vi "Test_InsertAndRemoveViewModel_NoError.vi"(8 "error in (no error)":errorcluster, 11 "TestCase in":refnum<class "TestIViewModel.lvclass">) -> (0 "error out":errorcluster, 3 "TestCase out":refnum<class "TestIViewModel.lvclass">)   [LabVIEW 2017, in "TestIViewModel.lvclass"]
uses:
  TestIViewModel.lvclass
  Framework/IViewModel/IViewModel/IViewModel.lvclass
  C:/Git/mva-framework/Framework/IViewManager/IViewManager/IViewManager.lvclass
  C:/Program Files (x86)/National Instruments/LabVIEW 2017/vi.lib/ActorFramework/Actor/Actor.lvclass
  Doubles/ViewableDoubles/ViewableOne/ViewableOne.lvclass
  C:/Git/mva-framework/Framework/IViewable/IViewable/IViewable.lvclass
  Framework/IModel/IModel/IModel.lvclass
  Framework/Mediator/Mediator/Mediator.lvclass
  C:/Git/mva-framework/Framework/IMediator/IMediator/IMediator.lvclass
  Framework/IViewModel/IViewModel/IViewModel.lvclass/IViewModel.ctl
  Framework/IViewManager/IViewManager Messages/Launch Nested Views Msg/Launch Nested Views Msg.lvclass/Launch Nested Views Msg.ctl
  Framework/IViewManager/IViewManager/IViewManager.lvclass/IViewManager.ctl
  Framework/IViewable/IViewable Messages/Insert Front Panel Msg/Insert Front Panel Msg.lvclass/Insert Front Panel Msg.ctl
  <vilib>/ActorFramework/Message Enqueuer/Message Enqueuer.lvclass/Message Enqueuer.ctl
  Framework/IViewable/IViewable Messages/Close Front Panel Msg/Close Front Panel Msg.lvclass/Close Front Panel Msg.ctl
  Framework/IViewManager/IViewManager Messages/Launch Nested Views Msg/Pack Launch Nested Views Msg.vi
  Framework/IViewManager/IViewManager/Write Startup Launch Nested Views Msg.vi
  <vilib>/ActorFramework/Message Enqueuer/Enqueue.vi
  Framework/IViewable/IViewable Messages/Insert Front Panel Msg/Insert Front Panel Msg.lvclass
  C:/Program Files (x86)/National Instruments/LabVIEW 2017/vi.lib/ActorFramework/Message/Message.lvclass
  Framework/IViewable/IViewable Messages/Close Front Panel Msg/Close Front Panel Msg.lvclass
  <vilib>/ActorFramework/Stop Msg/Stop Msg.lvclass
  <vilib>/ActorFramework/Message Priority Queue/Priority Enqueue.vi
  Framework/IViewable/IApplicationStyle/IApplicationStyle.lvclass
  Framework/IViewManager/IViewManager Messages/Launch Nested Views Msg/Launch Nested Views Msg.lvclass
  <vilib>/ActorFramework/Actor/Actor.lvclass
  Framework/IViewable/ProtectedSubpanel/ProtectedSubpanel.lvclass
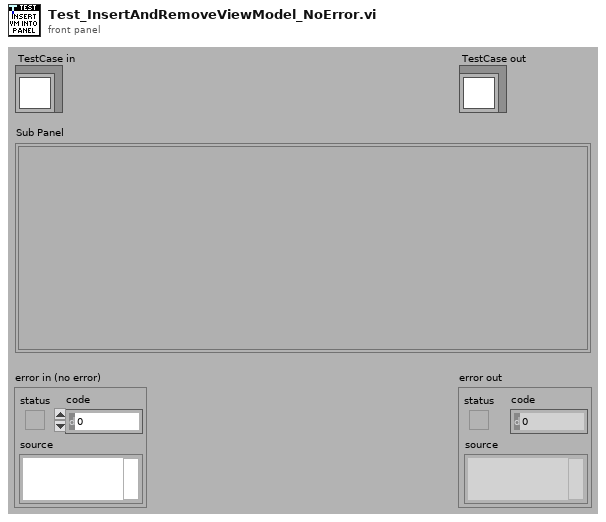
[diagram p1: front panel]
types:
  T1 = typedef "IViewable.lvlib/ProtectedSubpanel.lvclass/Protected Subpanel Reference.ctl" = refnum<data-value>
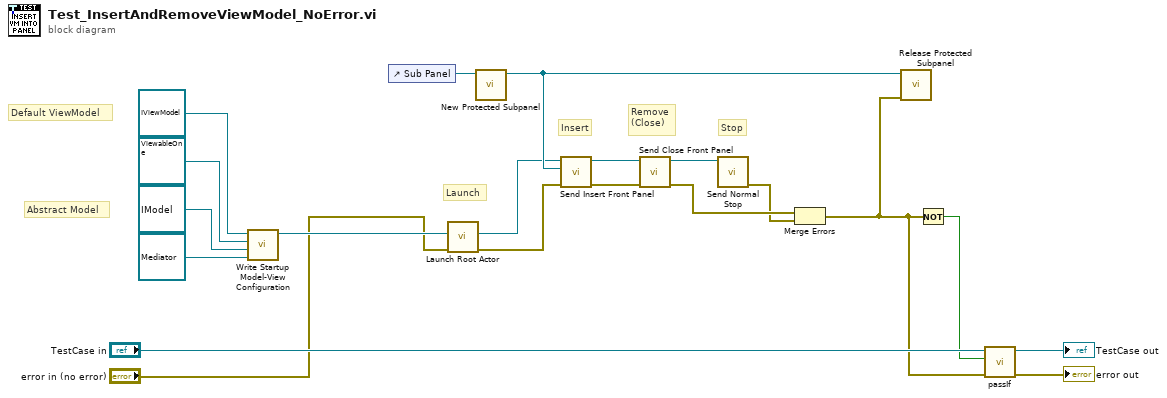
[diagram p0: block diagram]
diagram:
  # "Remove\n(Close)"
  # "Insert"
  # "Stop"
  # "Launch"
  # "Abstract Model"
  # "Default ViewModel"
  n1 = call "Write Startup Model-View Configuration.vi"("Mediator Type"=refnum<class "Mediator.lvclass"> refnum ("Mediator"), "Model Type"=refnum<class "IModel.lvclass"> refnum ("Model"), "Startup View Configuration"=refnum<class "ViewableOne.lvclass"> refnum, "IViewModel In"=refnum<class "IViewModel.lvclass"> refnum) -> ("IViewModel Out"=w12:refnum<class "IViewModel.lvclass">)  [unwired: 7 in]
  n2 = control-ref of="Sub Panel"() -> (w10:refnum<vi>)
  n3 = call <vilib>:"Launch Root Actor.vi"("error in (no error)"="error in (no error)", "Actor"=w12) -> ("error out"=w6:errorcluster, "Actor's Enqueuer"=w7:refnum<class "Message Enqueuer.lvclass">)  [unwired: 8 in]
  n4 = call "New Protected Subpanel.vi"("SubPnl Refnum"=w10) -> ("Protected Subpanel"=w9:T1)  [unwired: 9 in, 1 out]
  n5 = call "Send Insert Front Panel.vi"("error in (no error)"=w6, "Protected Subpanel"=w9, "Message Enqueuer"=w7) -> ("error out"=w5:errorcluster, "Message Enqueuer out"=w1:refnum<class "Message Enqueuer.lvclass">)  [unwired: 7 in]
  n6 = call "Send Close Front Panel.vi"("error in (no error)"=w5, "Message Enqueuer"=w1) -> ("error out"=w4:errorcluster, "Message Enqueuer out"=w2:refnum<class "Message Enqueuer.lvclass">)  [unwired: 8 in]
  n7 = call <vilib>:"Send Normal Stop.vi"("Message Enqueuer"=w2) -> ("error out"=w3:errorcluster)  [unwired: 10 in]
  n8 = Merge Errors(w4, w3) -> (w8:errorcluster)
  n9 = call "Release Protected Subpanel.vi"("error in (no error)"=w8, "Protected Subpanel"=w9) -> ()  [unwired: 9 in, 1 out]
  n10 = Not(x=w8) -> (.not. x?=w17:bool)
  n11 = call-dynamic "passIf.vi"("error in (no error)"=w8, "pass"=w17, "TestCase in"="TestCase in") -> ("error out"=→"error out":errorcluster, "TestCase out"=→"TestCase out":refnum<class "TestIViewModel.lvclass">)  [unwired: 7 in]
